vi "value by encoders to santimeters for back (SubVI).vi"(8 "error in (no error)":errorcluster, 11 "range in":dbl format="%#_13g") -> (0 "error out":errorcluster, 3 "value >= range":bool, 5 "curret value 2":i32)   [LabVIEW 2017]
uses:
  <vilib>/myRIO/Common/Instrument Driver Framework/myRIO v1.0/Encoder/typedefs/Encoder Signal Mode.ctl
  <vilib>/myRIO/Common/Instrument Driver Framework/myRIO v1.0/Encoder/typedefs/Encoder Channels Enum.ctl
  <vilib>/myRIO/Common/Instrument Driver Framework/Utilities/typedefs/Generic FPGA Reference.ctl
  <vilib>/myRIO/Common/Instrument Driver Framework/Utilities/typedefs/myRIO v1.0 Reference.ctl
  <vilib>/myRIO/Common/Instrument Driver Framework/Utilities/typedefs/Hardware Version Enum.ctl
  <vilib>/myRIO/Common/Instrument Driver Framework/Utilities/typedefs/myRIO Generic Hardware Reference.ctl
  <vilib>/myRIO/Instrument Drivers/Onboard IO/Encoder/typedefs/Encoder Reference.ctl
  <vilib>/myRIO/Instrument Drivers/Onboard IO/Encoder/Encoder.lvlib
  <vilib>/myRIO/Instrument Drivers/Onboard IO/Encoder/vis/Read.vi
  <vilib>/myRIO/Common/Instrument Driver Framework/myRIO v1.0/Encoder/typedefs/Encoder Configuration v1.0.ctl
  <vilib>/userdefined/High Color/nirio_resource_hc.ctl
  <vilib>/myRIO/Common/Instrument Driver Framework/myRIO v1.0/Encoder/vis/myRIO v1.1 Open Encoder.vi
  <vilib>/myRIO/Common/Instrument Driver Framework/myRIO v1.0/Encoder/vis/myRIO v1.0 Configure Encoder.vi
  <vilib>/myRIO/Instrument Drivers/Onboard IO/Encoder/vis/myRIO Encoder Open.xnode
  <vilib>/myRIO/Common/Instrument Driver Framework/Utilities/vis/Is FPGA Ref Available.vi
  <vilib>/myRIO/Express VI/Onboard IO/Encoder/Encoder Express VI.xnode
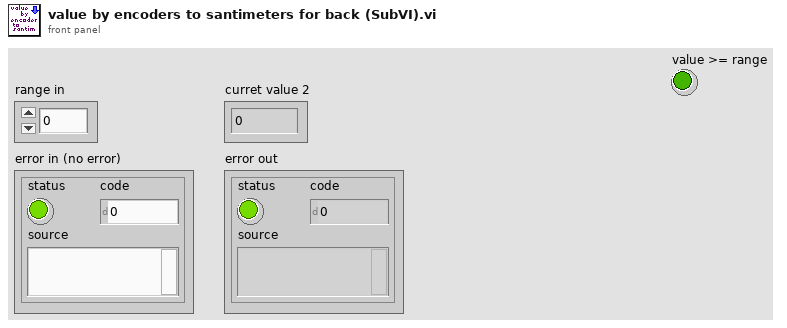
[diagram p1: front panel]
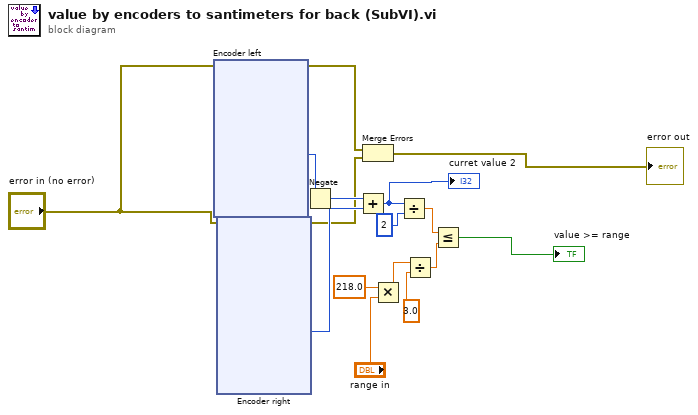
[diagram p0: block diagram]
diagram:
  n1 = xnode "Encoder left"("error in (no error)"="error in (no error)") -> ("Counter Value"=w4:i32, "error out"=w2:errorcluster)  [unwired: 1 in, 2 out]
  n2 = xnode "Encoder right"("error in (no error)"="error in (no error)") -> ("Counter Value"=w5:i32, "error out"=w3:errorcluster)  [unwired: 1 in, 2 out]
  n3 = Negate(x=w4) -> (-x=w9:i32)
  n4 = Add(x=w9, y=w5) -> (x+y=w10:i32)
  "curret value 2" <- w10
  n5 = Merge Errors(w2, w3) -> (→"error out":errorcluster)
  n6 = Multiply(x=218.0, y="range in") -> (x*y=w13:dbl)
  n7 = Divide(x=w10, y=2) -> (x/y=w7:dbl)
  n8 = Divide(x=w13, y=3.0) -> (x/y=w12:dbl)
  n9 = Less Or Equal?(x=w7, y=w12) -> (x <= y?=→"value >= range":bool)
